vi "subSystem1-1.vi"() -> ()   [LabVIEW 2012, in "GUILib.lvlib"]
doc: "an example for a sub-system"
uses:
  GUILib.lvlib
  GUILib.userEventsMainType.ctl
  GUILib.simpleNumeric.ctl
  GUILib.basicNumeric.ctl
  UtilityLib/UtilityLib.valueStatus.ctl
  UtilityLib/UtilityLib.lvlib
panel:
  in  "stop":bool
  in  "configure":bool
  in  "name3Ctl":T1 {"nom" step=22.0}
  in  "name2Ctl":T1 {"nom" step=22.0}
  in  "name1Ctl":T1 {"nom" step=22.0}
  in  "dummy":bool
  in  "parentSystem":bool
  in  "name3":bool=TRUE
  in  "name2":bool=TRUE
  in  "name1":bool=TRUE
  in  "userEvent":refnum<user-event>
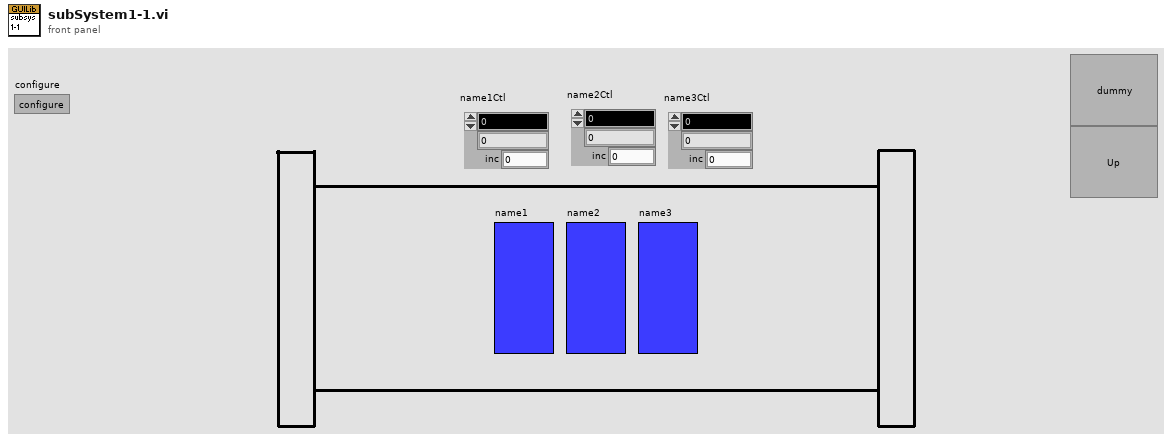
[diagram p1: front panel]
types:
  T1 = typedef "GUILib.lvlib/GUILib.simpleNumeric.ctl" = cluster{"nom":T2, "act":dbl, "inc":dbl}
  T2 = typedef "GUILib.lvlib/GUILib.basicNumeric.ctl" = dbl
  T3 = typedef "UtilityLib.lvlib/UtilityLib.valueStatus.ctl" = enum16{"no info available", "stand by/off", "on", "warning", "alarm/malfunction", "not implemented", "user action required", "important information", "system default", "control default", "indicator default", "button default"}
  T4 = typedef "GUILib.lvlib/GUILib.userEventsMainType.ctl" = cluster{"data":string, "dataType":i32}
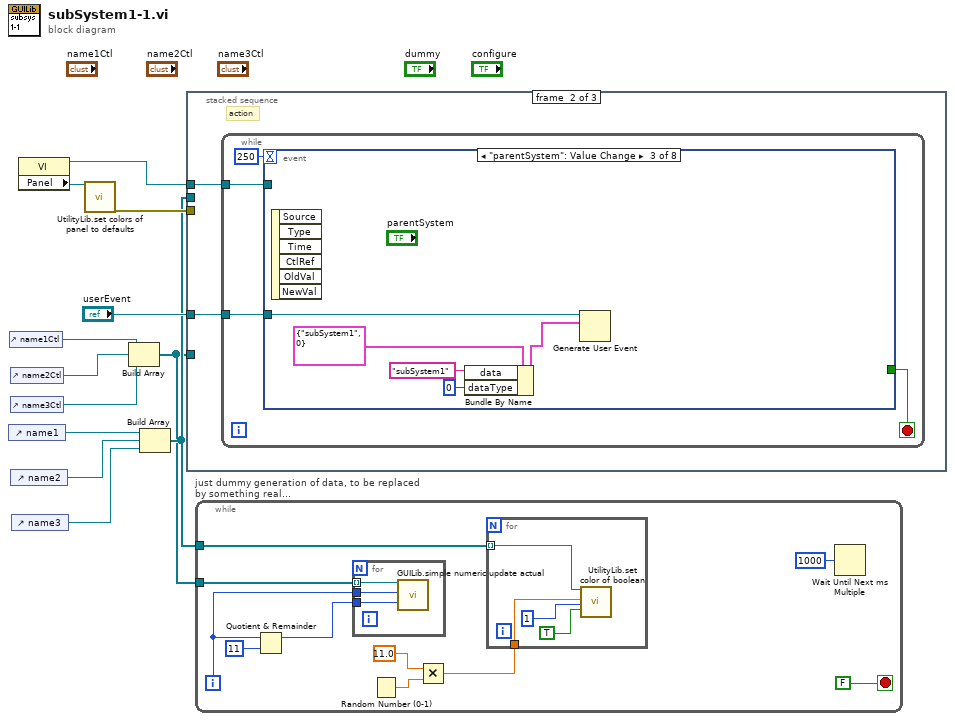
[diagram p0: block diagram]
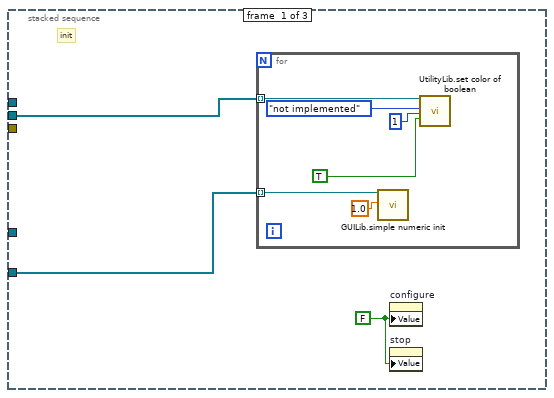
[diagram p2: hidden frame]
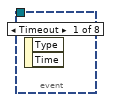
[diagram p3: hidden frame]
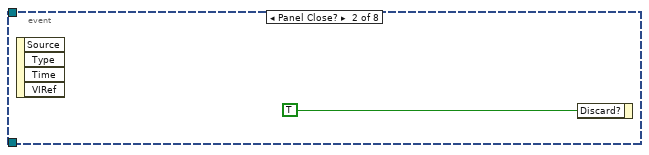
[diagram p4: hidden frame]
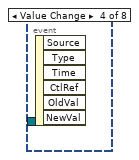
[diagram p5: hidden frame]
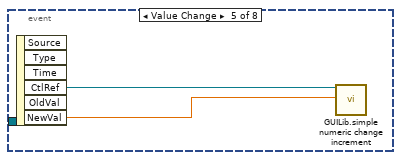
[diagram p6: hidden frame]
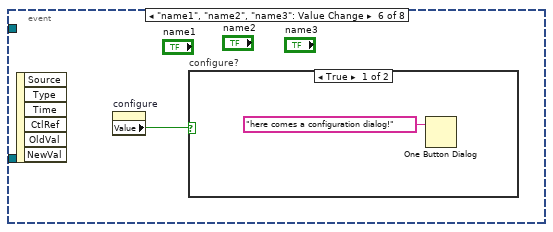
[diagram p7: hidden frame]
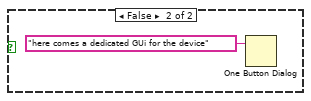
[diagram p8: hidden frame]
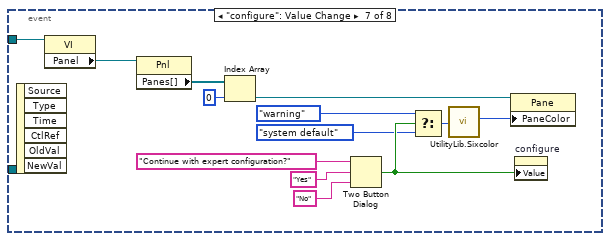
[diagram p9: hidden frame]
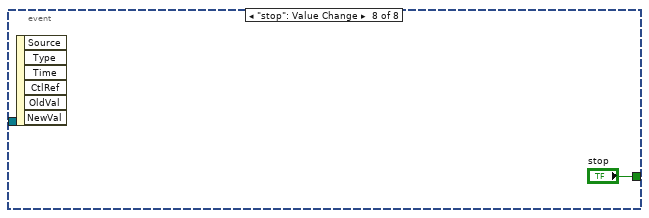
[diagram p10: hidden frame]
diagram:
  n1 = control-ref of="name1"() -> (w6:refnum<vi>)
  n2 = control-ref of="name1Ctl"() -> (w4:refnum<vi>)
  n3 = control-ref of="name2Ctl"() -> (w3:refnum<vi>)
  n4 = control-ref of="name3Ctl"() -> (w2:refnum<vi>)
  n5 = control-ref of="name2"() -> (w7:refnum<vi>)
  n6 = control-ref of="name3"() -> (w8:refnum<vi>)
  n7 = property on="Property Node" class="VI"() -> (reference out=w10:refnum<vi>, "Panel"=w11:refnum<vi>)  [unwired: 2 in, 1 out]
  n8 = call "UtilityLib.set colors of panel to defaults.vi"("Front Panel"=w11) -> ("error out"=w9:errorcluster)  [unwired: 18 in]
  n9 = Build Array(w4, w3, w2) -> (w1:refnum<vi>[])
  n10 = Build Array(w6, w7, w8) -> (w5:refnum<vi>[])
  n11 = stacked-sequence {
    tunnel: "userEvent" -> [_ w23 _]
    tunnel: w10 -> [_ w22 _]
    tunnel: w9 -> [_ _ _]
    tunnel: w5 -> [w15 _ _]
    tunnel: w1 -> [w14 _ _]
    frame #0 {
      w13 = FALSE ("configure")
      # "init"
      n12 = for {
        tunnel: w15 -> [w18] mode=indexing
        tunnel: w14 -> [w16] mode=indexing
        n13 = call "GUILib.simple numeric init.vi"("ctlRef"=w16, "increment"=1.0) -> ()  [unwired: 16 in, 2 out]
        n14 = call "UtilityLib.set color of boolean.vi"("button"=w18, "valueStatus"=UtilityLib.valueStatus."not implemented", "nOfPair (0)"=1, "setTRUEColor (FALSE)"=TRUE) -> ()  [unwired: 15 in, 1 out]
      }
      n15 = property on="configure" class="Bool (strict)"("Value"=w13) -> ()  [unwired: 2 in, 2 out]
      n16 = property on="stop" class="Bool (strict)"("Value"=w13) -> ()  [unwired: 2 in, 2 out]
    }
    frame #1 {
      # "action"
      n17 = while {
        tunnel: w23 -> [w27]
        tunnel: w22 -> [w25]
        stop <- w24 stop-if-true
        n18 = event shown="[2] \"parentSystem\": Value Change" {
          selector: _ -> [_ _ _ _ _ _ _ _]
          dyn-events: _ -> [_ _ _ _ _ _ _ _]
          timeout: 250 -> [_ _ _ _ _ _ _ _]
          tunnel: w27 -> [_ _ w33 _ _ _ _ _]
          tunnel: w25 -> [_ _ _ _ _ _ w50 _]
          tunnel: [_ _ _ _ _ _ _ "stop"] -> w24
          event Timeout {
            n19 = event-data() -> ()  [unwired: 1 in, 2 out]
          }
          event Panel Close? {
            n20 = event-data() -> ()  [unwired: 1 in, 4 out]
            n21 = event-data ("Event Filter Node")("Discard?"=TRUE) -> ()  [unwired: 1 in, 1 out]
          }
          event "parentSystem": Value Change {
            n22 = event-data() -> ()  [unwired: 1 in, 6 out]
            n23 = Bundle By Name(cluster=T4 {"data"="subSystem1", "dataType"=0} ("userEventsMain"), "data"="subSystem1", "dataType"=0) -> (w31:T4)
            n24 = Generate User Event(user event=w33, event data cluster=w31) -> ()  [unwired: 1 in, 2 out]
          }
          event Value Change {
            n25 = event-data() -> ()  [unwired: 1 in, 6 out]
          }
          event Value Change {
            n26 = event-data() -> ("CtlRef"=w35:refnum<vi>, "NewVal"=w34:dbl)  [unwired: 1 in, 4 out]
            n27 = call "GUILib.simple numeric change increment.vi"("ctlRef"=w35, "increment"=w34) -> ()  [unwired: 16 in, 2 out]
          }
          event "name1", "name2", "name3": Value Change {
            n28 = event-data() -> ()  [unwired: 1 in, 6 out]
            n29 = property on="configure" class="Bool (strict)"() -> ("Value"=w36:bool)  [unwired: 2 in, 2 out]
            n30 = case "configure?" shown="True" w36 {
              frame True {
                n31 = One Button Dialog(message="here comes a configuration dialog!") -> ()  [unwired: 1 in, 1 out]
              }
              frame False {
                n32 = One Button Dialog(message="here comes a dedicated GUi for the device") -> ()  [unwired: 1 in, 1 out]
              }
            }
          }
          event "configure": Value Change {
            n33 = event-data() -> ()  [unwired: 1 in, 6 out]
            n34 = property on="Property Node" class="VI"(reference=w50) -> ("Panel"=w49:refnum<vi>)  [unwired: 1 in, 2 out]
            n35 = property on="Property Node" class="Pnl"(reference=w49) -> ("Panes[]"=w48:refnum<vi>[])  [unwired: 1 in, 2 out]
            n36 = Index Array(array=w48, index=0) -> (element=w46:refnum<vi>)
            n37 = Two Button Dialog(message="Continue with expert configuration?", 1:"No" ("F button name (\"Cancel\")"), 2:"Yes" ("T button name (\"OK\")")) -> (T button?=w45:bool)
            n38 = Select(t=UtilityLib.valueStatus."warning", s=w45, f=UtilityLib.valueStatus."system default" ("valueStatus")) -> (s? t:f=w43:T3)
            n39 = call "UtilityLib.Sixcolor.vi"("State"=w43) -> ("elementBackground"=w44:u32)  [unwired: 2 in, 3 out]
            n40 = property on="Property Node" class="Pane"(reference=w46, "PaneColor"=w44) -> ()  [unwired: 1 in, 2 out]
            n41 = property on="configure" class="Bool (strict)"("Value"=w45) -> ()  [unwired: 2 in, 2 out]
          }
          event "stop": Value Change {
            n42 = event-data() -> ()  [unwired: 1 in, 6 out]
          }
        }
      }
    }
    frame #2 {
      # "deinit"
    }
  }
  n43 = while "just dummy generation of data, to be replaced by something real..." {
    tunnel: w5 -> [w54]
    tunnel: w1 -> [w53]
    i -> [w59]
    stop <- FALSE stop-if-true
    n44 = Quotient & Remainder(x=w59, y=11) -> (x-y*floor(x/y)=w58:i32)  [unwired: 1 out]
    n45 = for {
      tunnel: w59 -> [w65]
      tunnel: w58 -> [w64]
      tunnel: w53 -> [w63] mode=indexing
      n46 = call "GUILib.simple numeric update actual.vi"("ctlRef"=w63, "actualValue"=w65, "valueStatus"=w64) -> ()  [unwired: 15 in, 2 out]
    }
    n47 = Random Number (0-1)() -> (number: 0 to 1=w57:dbl)
    n48 = Multiply(x=11.0, y=w57) -> (x*y=w55:dbl)
    n49 = for {
      tunnel: w55 -> [w67]
      tunnel: w54 -> [w66] mode=indexing
      n50 = call "UtilityLib.set color of boolean.vi"("button"=w66, "valueStatus"=w67, "nOfPair (0)"=1, "setTRUEColor (FALSE)"=TRUE) -> ()  [unwired: 15 in, 1 out]
    }
    n51 = Wait Until Next ms Multiple(millisecond multiple=u32 1000) -> ()  [unwired: 1 out]
  }
